vi "主面板.vi"() -> ()   [LabVIEW 2018]
uses:
  <vilib>/Utility/file.llb/Read Delimited Spreadsheet (string).vi
panel:
  out "状态栏2":string
  out "状态栏1":string
  out "字符串":string
  out "时间":string
  out "日期":string
  out "气候":string
  out "气温":string
  out "表格":string[][](table)
  in  "更新":bool
  in  "消毒":bool
  in  "取":bool
  in  "存":bool
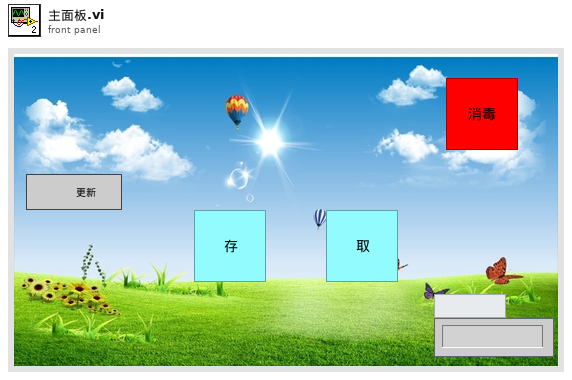
[diagram p1: front panel]
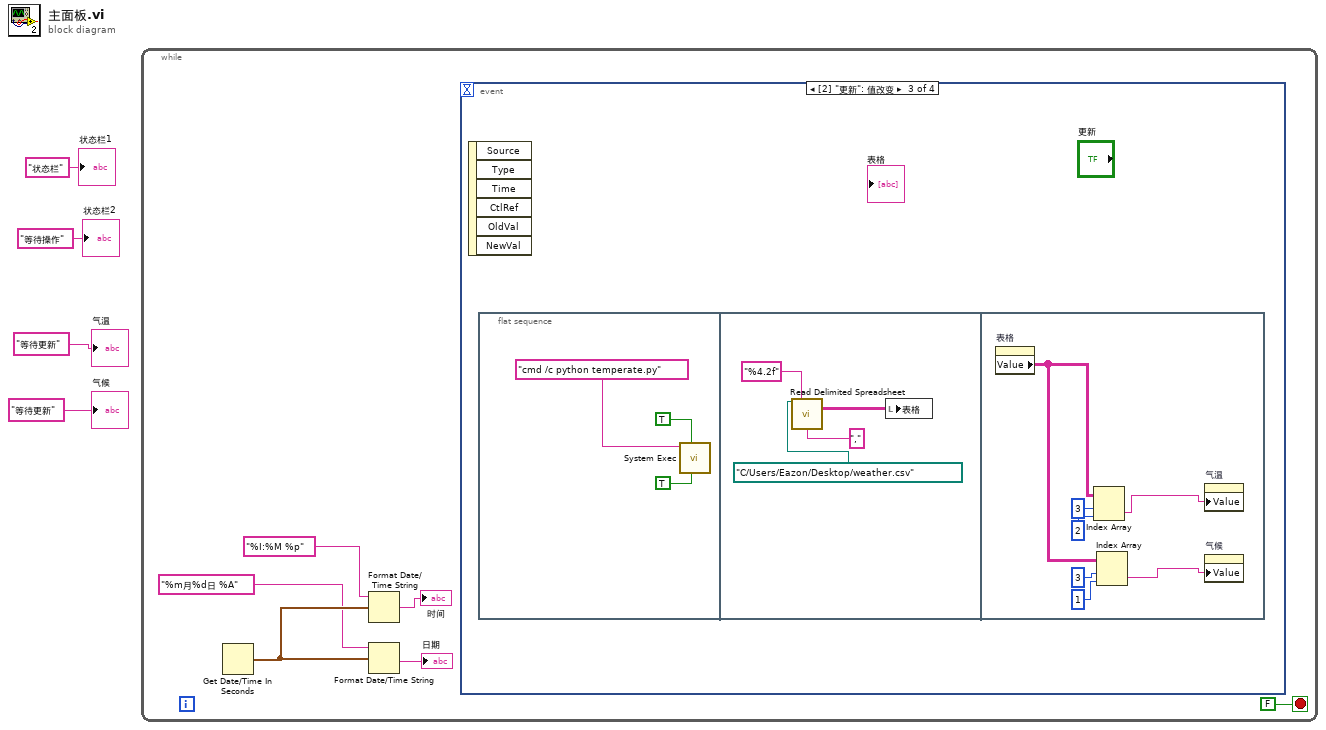
[diagram p0: block diagram]
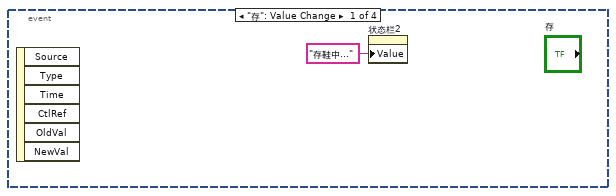
[diagram p2: hidden frame]
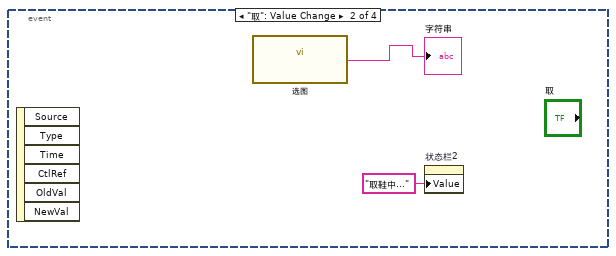
[diagram p3: hidden frame]
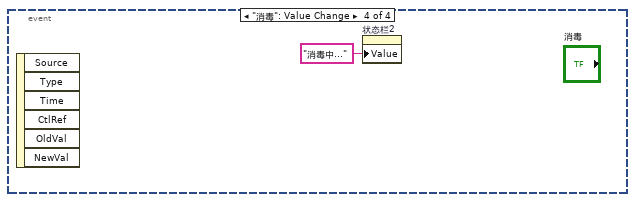
[diagram p4: hidden frame]
diagram:
  n1 = while {
    stop <- FALSE stop-if-true
    n2 = Get Date/Time In Seconds() -> (seconds since 1Jan1904=w9:timestamp)
    n3 = Format Date/Time String(time format string (%c)="%I:%M %p" ("时间格式字符串(%c)"), seconds (now)=w9) -> (date/time string=→"时间":string)  [unwired: 1 in]
    n4 = Format Date/Time String(time format string (%c)="%m月%d日 %A" ("时间格式字符串(%c)"), seconds (now)=w9) -> (date/time string=→"日期":string)  [unwired: 1 in]
    n5 = event shown="[2] \"更新\": 值改变" {
      selector: _ -> [_ _ _ _]
      dyn-events: _ -> [_ _ _ _]
      timeout: _ -> [_ _ _ _]
      event "存": Value Change {
        n6 = event-data() -> ()  [unwired: 1 in, 6 out]
        n7 = property on="状态栏2" class="Str"("Value"="存鞋中..." ("状态栏2")) -> ()  [unwired: 2 in, 2 out]
      }
      event "取": Value Change {
        n8 = event-data() -> ()  [unwired: 1 in, 6 out]
        n9 = call "选图.vi"() -> ("选鞋数据"=→"字符串":string)  [unwired: 1 in]
        n10 = property on="状态栏2" class="Str"("Value"="取鞋中..." ("状态栏2")) -> ()  [unwired: 2 in, 2 out]
      }
      event "更新": Value Change {
        n11 = event-data() -> ()  [unwired: 1 in, 6 out]
        n12 = flat-sequence {
          frame #0 {
            n13 = call <vilib>:"System Exec.vi"("run minimized? (F)"=TRUE, "wait until completion? (T)"=TRUE, "command line"="cmd /c python temperate.py") -> ()  [unwired: 5 in, 4 out]
          }
          frame #1 {
            n14 = call-poly <vilib>:"Read Delimited Spreadsheet.vi"("file path (dialog if empty)"=path "C:/Users/Eazon/Desktop/weather.csv", "format (%s)"="%4.2f" ("format (%.3f)"), "delimiter (\\t)"="," ("delimiter (\\t)")) -> ("all rows"=w20:string[][])  [unwired: 7 in, 5 out]
            n15 = local write "表格"(w20) -> ()
          }
          frame #2 {
            n16 = property on="表格" class="Tbl (严格)"() -> ("Value"=w25:string[][])  [unwired: 2 in, 2 out]
            n17 = Index Array(array=w25, index (row)=3 ("索引 (行)"), index (col)=2 ("禁用的索引 (列)")) -> (element=w26:string)
            n18 = Index Array(array=w25, index (row)=3 ("索引 (行)"), index (col)=1 ("禁用的索引 (列)")) -> (element=w27:string)
            n19 = property on="气温" class="Str"("Value"=w26) -> ()  [unwired: 2 in, 2 out]
            n20 = property on="气候" class="Str"("Value"=w27) -> ()  [unwired: 2 in, 2 out]
          }
        }
      }
      event "消毒": Value Change {
        n21 = event-data() -> ()  [unwired: 1 in, 6 out]
        n22 = property on="状态栏2" class="Str"("Value"="消毒中..." ("状态栏2")) -> ()  [unwired: 2 in, 2 out]
      }
    }
  }
  "气温" <- "等待更新" ("天气情况")
  "气候" <- "等待更新" ("天气情况")
  "状态栏2" <- "等待操作" ("状态栏2")
  "状态栏1" <- "状态栏" ("状态栏1")
